vi "Writestatus.vi"(8 "error in (no error)":errorcluster, 10 "status":T1, 11 "object in":refnum<class "status Message.lvclass">) -> (0 "error out":errorcluster, 3 "object out":refnum<class "status Message.lvclass">)   [LabVIEW 2018, in "ClientMessaging.lvlib" / "status Message.lvclass"]
uses:
  status Message.lvclass
  Status Content.ctl
  status Message.lvclass/status Message.ctl
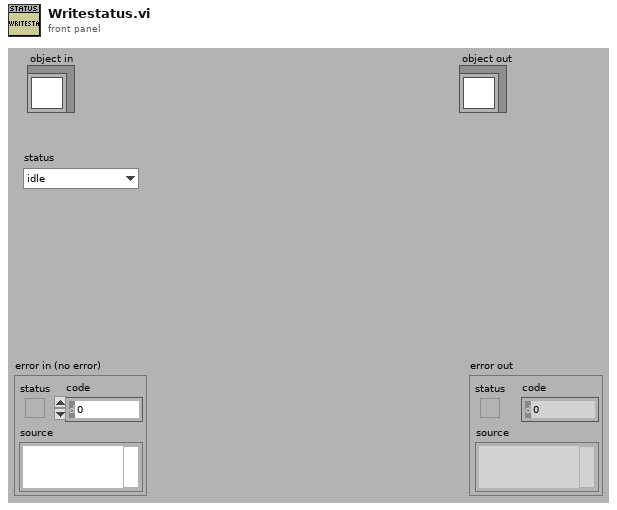
[diagram p1: front panel]
types:
  T1 = typedef "ClientMessaging.lvlib/status Message.lvclass/Status Content.ctl" = enum16{"idle", "busy", "starting"}
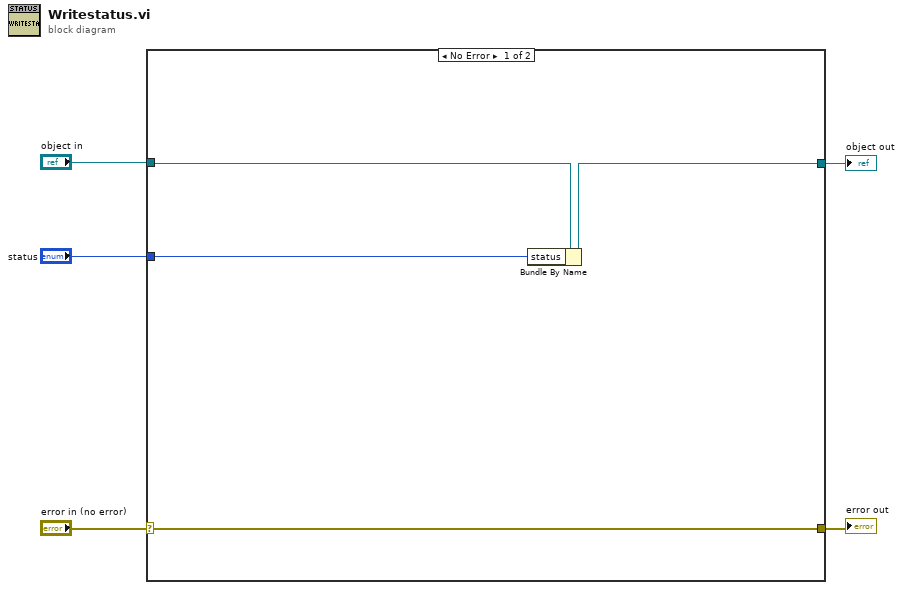
[diagram p0: block diagram]
diagram:
  n1 = case shown="No Error" "error in (no error)" {
    selector: "error in (no error)" -> [w8 w11]
    tunnel: [w8 w11] -> w4
    tunnel: [w6 w10] -> w2
    tunnel: "object in" -> [w7 w10]
    tunnel: "status" -> [w9 _]
    frame No Error {
      n2 = Bundle By Name(cluster=w7, "status"=w9) -> (w6:refnum<class "status Message.lvclass">)
    }
    frame Error {
    }
  }
  "error out" <- w4
  "object out" <- w2
